vi "Insert.vi"(8 "error in (no error)":errorcluster, 10 "VI Ref":refnum<vi>, 11 "subpanel_abstract in":refnum<class "subpanel (abstract).lvclass">) -> (0 "error out":errorcluster, 3 "subpanel_abstract out":refnum<class "subpanel (abstract).lvclass">)   [LabVIEW 2023, in "GUI.lvlib" / "subpanel (abstract).lvclass"]
uses:
  subpanel (abstract).lvclass
  <vilib>/Utility/miscctls.llb/LVPointTypeDef.ctl
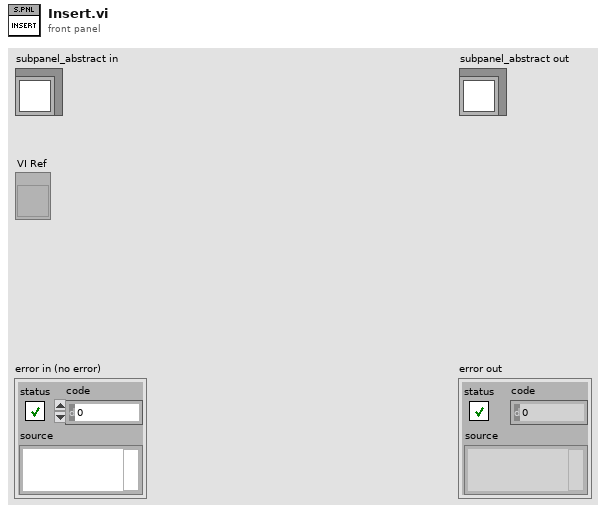
[diagram p1: front panel]
types:
  T1 = typedef "LVPointTypeDef.ctl" = cluster{"Horizontal":i16, "Vertical":i16}
  T2 = enum16{"Always On", "Always Off", "Off While Running"}
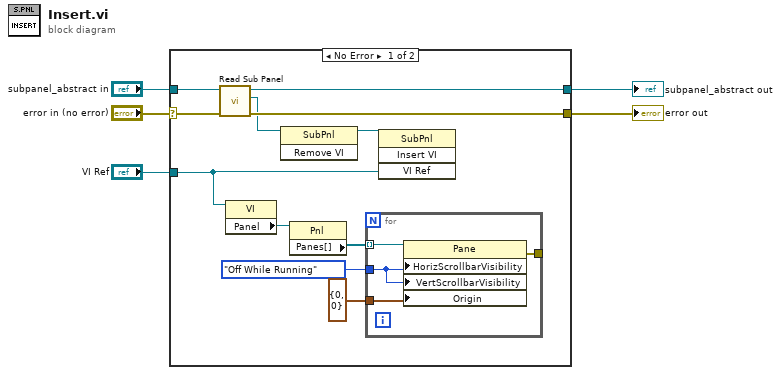
[diagram p0: block diagram]
diagram:
  n1 = case shown="No Error" "error in (no error)" {
    selector: "error in (no error)" -> [w15 w22]
    tunnel: [w13 w22] -> w4
    tunnel: [w14 w21] -> w2
    tunnel: "subpanel_abstract in" -> [w16 w21]
    tunnel: "VI Ref" -> [w10 _]
    frame No Error {
      n2 = call-dynamic "Read Sub Panel.vi"("error in (no error)"=w15, "subpanel_abstract in"=w16) -> ("error out"=w13:errorcluster, "Sub Panel"=w12:refnum<vi>, "subpanel_abstract out"=w14:refnum<class "subpanel (abstract).lvclass">)  [unwired: 7 in]
      n3 = property class="VI"(reference=w10) -> ("Panel"=w9:refnum<vi>)  [unwired: 1 in, 2 out]
      n4 = invoke class="SubPnl" method="Remove VI"(reference=w12) -> (reference out=w11:refnum<vi>)  [unwired: 2 in, 2 out]
      n5 = property class="Pnl"(reference=w9) -> ("Panes[]"=w8:refnum<vi>[])  [unwired: 1 in, 2 out]
      n6 = for {
        tunnel: w8 -> [w20] mode=indexing
        tunnel: T2."Off While Running" ("Horizontal Scrollbar Visibility") -> [w19]
        tunnel: [w18] -> _
        tunnel: T1 {"Horizontal"=0, "Vertical"=0} ("Origin") -> [w17]
        n7 = property class="Pane"(reference=w20, "HorizScrollbarVisibility"=w19, "VertScrollbarVisibility"=w19, "Origin"=w17) -> (error out=w18:errorcluster)  [unwired: 1 in, 1 out]
      }
      n8 = invoke class="SubPnl" method="Insert VI"(reference=w11, "VI Ref"=w10) -> ()  [unwired: 2 in, 4 out]
    }
    frame Error {
    }
  }
  "error out" <- w4
  "subpanel_abstract out" <- w2
